vi "PSU RANGE CALC.vi"() -> ()   [LabVIEW 2011]
panel:
  in  "low cuttoff":dbl
  in  "window":dbl
  out "High":dbl
  out "Low":dbl
  in  "multiplier":dbl
  out "Multiplier":string
  out "Lower Cutoff":dbl
  out "Window (Delta-T)":dbl
  in  "High speed (m/s)":dbl=3000.0
  in  "Low speed (m/s)":dbl=2000.0
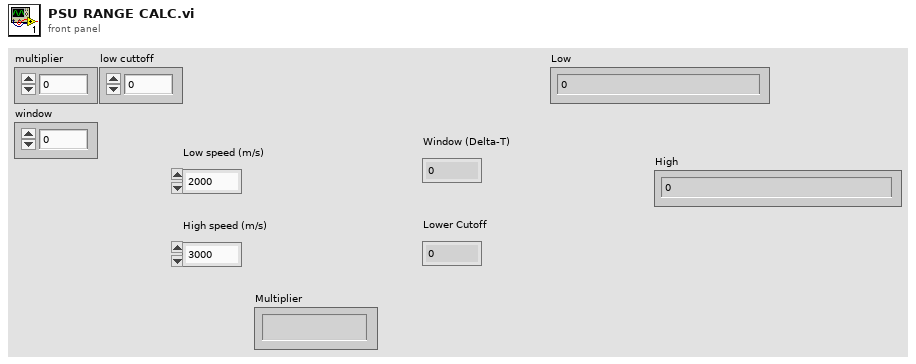
[diagram p1: front panel]
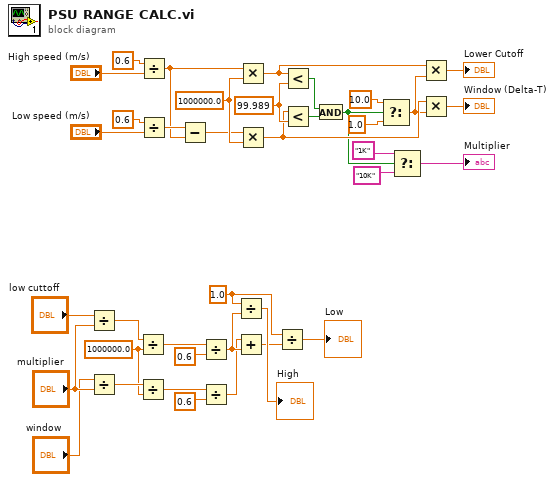
[diagram p0: block diagram]
diagram:
  w11 = 1.0 ("x")
  w14 = 1000000.0 ("y")
  w30 = 99.989
  w32 = 1000000.0 ("y")
  n1 = Divide(x="low cuttoff", y="multiplier") -> (x/y=w15:dbl)
  n2 = Divide(x="window", y="multiplier") -> (x/y=w18:dbl)
  n3 = Divide(x=w15, y=w14) -> (x/y=w12:dbl)
  n4 = Divide(x=w18, y=w14) -> (x/y=w7:dbl)
  n5 = Divide(x=0.6, y="High speed (m/s)") -> (x/y=w33:dbl)
  n6 = Divide(x=0.6, y="Low speed (m/s)") -> (x/y=w34:dbl)
  n7 = Subtract(x=w34, y=w33) -> (x-y=w31:dbl)
  n8 = Divide(x=w12, y=0.6) -> (x/y=w9:dbl)
  n9 = Divide(x=w7, y=0.6) -> (x/y=w6:dbl)
  n10 = Divide(x=w11, y=w9) -> (x/y=→"High":dbl)
  n11 = Add(x=w6, y=w9) -> (x+y=w5:dbl)
  n12 = Multiply(x=w33, y=w32) -> (x*y=w24:dbl)
  n13 = Multiply(x=w31, y=w32) -> (x*y=w25:dbl)
  n14 = Divide(x=w11, y=w5) -> (x/y=→"Low":dbl)
  n15 = Less?(x=w24, y=w30) -> (x < y?=w29:bool)
  n16 = Less?(x=w25, y=w30) -> (x < y?=w28:bool)
  n17 = And(x=w29, y=w28) -> (x .and. y?=w20:bool)
  n18 = Select(t=10.0, s=w20, f=1.0) -> (s? t:f=w23:dbl)
  n19 = Select(t="1K", s=w20, f="10K") -> (s? t:f=→"Multiplier":string)
  n20 = Multiply(x=w24, y=w23) -> (x*y=→"Lower Cutoff":dbl)
  n21 = Multiply(x=w25, y=w23) -> (x*y=→"Window (Delta-T)":dbl)
